vi "))Channel.vi"(0 "channel in":T3, 1 "packet":string, 2 "This VI":refnum<vi>, 5 "channelOp":T5, 7 "parms in":T2={"subchannel"=0, "size (0)"=0, "abort (F)"=FALSE, "timeout"=-1, "ack id (0)"=0, "last elt? (F)"=FALSE, "valid? (T)"=FALSE, "GUID"=""}, 11 "element in":T4, 12 "replacement":refnum<class "MessengerMBase.lvclass">, 13 "nonfull/empty":refnum<k4>, 14 "ackOcc":refnum<k4>) -> (3 "This VI out":refnum<vi>, 4 "channel out":T3, 6 "wait":bool, 8 "parms out":T1, 15 "element out":T4)   [LabVIEW 2019, in "MessengerM.lvlib"]
uses:
  MessengerM.lvlib
  Element.ctl
  ChannelOp.ctl
  ))Channel.ctl
  MessengerMBase/MessengerMBase.lvclass
  ParmsIn.ctl
  ParmsOut.ctl
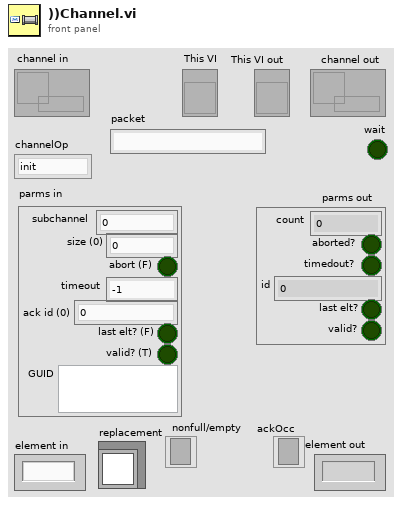
[diagram p1: front panel]
types:
  T1 = typedef "MessengerM.lvlib/ParmsOut.ctl" = cluster{"count":i32, "aborted?":bool, "timedout?":bool, "id":u32, "last elt?":bool, "valid?":bool}
  T2 = typedef "MessengerM.lvlib/ParmsIn.ctl" = cluster{"subchannel":i32, "size (0)":i32, "abort (F)":bool, "timeout":i32, "ack id (0)":u32, "last elt? (F)":bool, "valid? (T)":bool, "GUID":string}
  T3 = typedef "MessengerM.lvlib/))Channel.ctl" = refnum<queue>
  T4 = typedef "MessengerM.lvlib/Element.ctl" = string
  T5 = typedef "MessengerM.lvlib/ChannelOp.ctl" = enum16{"init", "write", "read", "wrtAck", "rdAck", "rdAck2", "probe"}
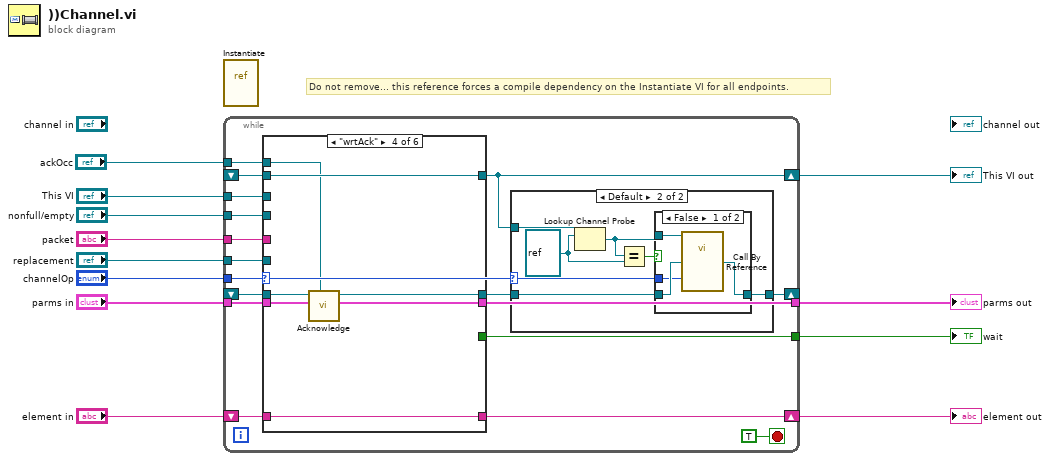
[diagram p0: block diagram]
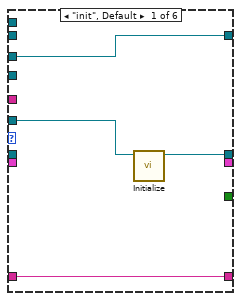
[diagram p4: hidden frame]
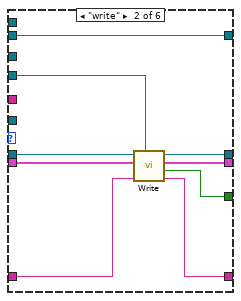
[diagram p5: hidden frame]
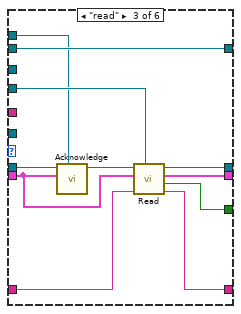
[diagram p6: hidden frame]
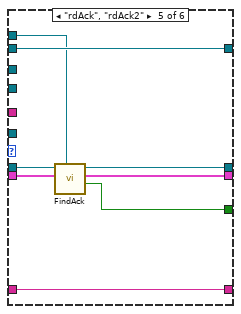
[diagram p7: hidden frame]
diagram:
  # "Do not remove... this reference forces a compile dependency on the Instantiate VI for all endpoints."
  n1 = vi-ref "Instantiate.vi"() -> ()  [unwired: 1 out]
  n2 = while {
    tunnel: "channelOp" -> [w19]
    shift-right: [w20] -> _
    shift-left: _ -> [w28]
    tunnel: [w25] -> w8
    tunnel: "This VI" -> [w24]
    shift-right: [w22] -> w10
    shift-left: _ -> [w23]
    shift-right: [w26] -> w5
    shift-left: "element in" -> [w27]
    tunnel: "nonfull/empty" -> [w18]
    tunnel: "replacement" -> [w17]
    tunnel: "ackOcc" -> [w16]
    tunnel: "packet" -> [w15]
    tunnel: "parms in" -> [w14]
    tunnel: [w13] -> w1
    stop <- TRUE stop-if-true
    n3 = case shown="\"wrtAck\"" w19 {
      tunnel: w28 -> [_ w55 w60 w73 w81 w84]
      tunnel: [w46 w54 w64 w70 w78 w84] -> w21
      tunnel: w27 -> [w45 w51 w63 w72 w80 w83]
      tunnel: [w45 w53 w62 w72 w80 w83] -> w26
      tunnel: [_ w48 w58 _ w76 _] -> w25
      tunnel: w24 -> [w44 _ _ _ _ _]
      tunnel: [w44 w52 w66 w71 w79 w82] -> w22
      tunnel: w23 -> [_ w52 w66 w71 w79 w82]
      tunnel: w18 -> [_ w50 w65 _ _ _]
      tunnel: w17 -> [w43 _ _ _ _ _]
      tunnel: w16 -> [_ _ w59 w69 w77 _]
      tunnel: w15 -> [_ _ _ _ _ _]
      tunnel: w14 -> [_ w49 w56 w68 w75 _]
      tunnel: [_ w47 w57 w67 w74 _] -> w13
      frame "init", Default {
        n4 = call-dynamic "Initialize.vi"("messengerMbase in"=w43) -> ("messengerMbase out"=w46:refnum<class "MessengerMBase.lvclass">)  [unwired: 10 in]
      }
      frame "write" {
        n5 = call-dynamic "Write.vi"("nonFull"=w50, "element in"=w51, "parms in"=w49, "messengerMbase in"=w55) -> ("element out"=w53:T4, "wait"=w48:bool, "parms out"=w47:T1, "messengerMbase out"=w54:refnum<class "MessengerMBase.lvclass">)  [unwired: 4 in]
      }
      frame "read" {
        n6 = call-dynamic "Acknowledge.vi"("ack"=w59, "parms in"=w56, "messengerMbase in"=w60) -> ("messengerMbase out"=w61:refnum<class "MessengerMBase.lvclass">)  [unwired: 7 in, 1 out]
        n7 = call-dynamic "Read.vi"("nonEmpty"=w65, "element in"=w63, "parms in"=w56, "messengerMbase in"=w61) -> ("element out"=w62:T4, "wait"=w58:bool, "parms out"=w57:T1, "messengerMbase out"=w64:refnum<class "MessengerMBase.lvclass">)  [unwired: 4 in]
      }
      frame "wrtAck" {
        n8 = call-dynamic "Acknowledge.vi"("ack"=w69, "parms in"=w68, "messengerMbase in"=w73) -> ("parms out"=w67:T1, "messengerMbase out"=w70:refnum<class "MessengerMBase.lvclass">)  [unwired: 7 in]
      }
      frame "rdAck", "rdAck2" {
        n9 = call-dynamic "FindAck.vi"("ack"=w77, "parms in"=w75, "messengerMbase in"=w81) -> ("wait"=w76:bool, "parms out"=w74:T1, "messengerMbase out"=w78:refnum<class "MessengerMBase.lvclass">)  [unwired: 6 in]
      }
      frame "probe" {
      }
    }
    n10 = case shown="Default" w19 {
      selector: w19 -> [_ w34]
      tunnel: w22 -> [_ w37]
      tunnel: w21 -> [w30 w36]
      tunnel: [w30 w35] -> w20
      frame "probe" {
      }
      frame Default {
        w31 = refnum<vi> refnum ("This VI")
        n11 = Lookup Channel Probe(0:w37, 1:w31) -> (9:w32:refnum<vi>)  [unwired: 1 in, 1 out]
        n12 = Equal?(x=w32, y=w31) -> (x = y?=w33:bool)
        n13 = case shown="False" w33 {
          tunnel: w32 -> [w41 _]
          tunnel: w36 -> [w40 w42]
          tunnel: [w39 w42] -> w35
          tunnel: w34 -> [w38 _]
          frame False {
            n14 = call-by-ref "?"(reference=w41, "channelOp"=w38, "mdata in"=w40) -> ("mdata out"=w39:refnum<class "MessengerMBase.lvclass">)  [unwired: 2 in, 2 out]
          }
          frame True {
          }
        }
      }
    }
  }
  "element out" <- w5
  "wait" <- w8
  "This VI out" <- w10
  "parms out" <- w1
